vi "표지판 가공.vi"(1 "Paramaters":T4 {"Preprocessing Options"."Deviation Factor" min=0.0; "Preprocessing Options"."Threshold Limits"."Upper value" format="%.2f"; "Preprocessing Options"."Threshold Limits"."Lower value" format="%.2f"; "Preprocessing Options"."Threshold Range"."Upper value" format="%.2f"; "Preprocessing Options"."Threshold Range"."Lower value" format="%.2f"; "Preprocessing Options"."# of Erosions" min=0; "Preprocessing Options"."Method" items=["Manual Threshold"=-1, "-"=-2, "Auto Threshold: Clustering"=0, "Auto Threshold: Entropy"=1, "Auto Threshold: Metric"=2, "Auto Threshold: Moments"=3, "Auto Threshold: Inter-class Variance"=4, "--"=-3, "Local Threshold: Niblack"=5, "Local Threshold: BG Correction"=6]; "Preprocessing Options"."Looking for" items=["Bright Objects", "Dark Objects"]; "Nearest Neighbor Options"."Method" items=["Nearest Neighbor", "K Nearest Neighbor", "Minimum Mean Distance"]; "Nearest Neighbor Options"."Metric" items=["Maximum", "Sum", "Euclidean"]; "Nearest Neighbor Options"."k" min=3}, 2 "File Path":path=path "C:/Users/SeongHyeon/Desktop/[Github]_GPS Team/labview_program/작업중인 모든 Vi, dll파일 모음/전체프로그램/Sub Vi/Sensor/Vision Reference/곡선2.clf", 3 "Classifier Session (optional)":T2, 4 "Image 2":T1) -> (0 "주차냐":bool)   [LabVIEW 2016]
uses:
  <vilib>/vision/Classification.llb/IMAQ Classifier Nearest Neighbor options.ctl
  <vilib>/vision/Classification.llb/IMAQ Classifier Session.ctl
  <vilib>/vision/Image Controls.llb/IMAQ Image.ctl
  <vilib>/vision/NI_Vision_Development_Module.lvlib
panel:
  out "Identification Score":sgl
  out "Image":T1(plugin-control)
  in  "ROI Descriptor (Particle Classification 1)":T5={"Global Rectangle"=[693, 212, 1098, 745], "Contours"=[{"ID"=enum."External", "Type"=3, "Coordinates"=[693, 212, 1098, 745]}]} {"Contours"."Type" items=["No Selection", "Point", "Line", "Rectangle", "Oval", "Polygon", "Freehand Region", "Annulus", "Unused2", "Unused3", "Broken Line", "Freehand Line", "Rotated Rectangle"]}
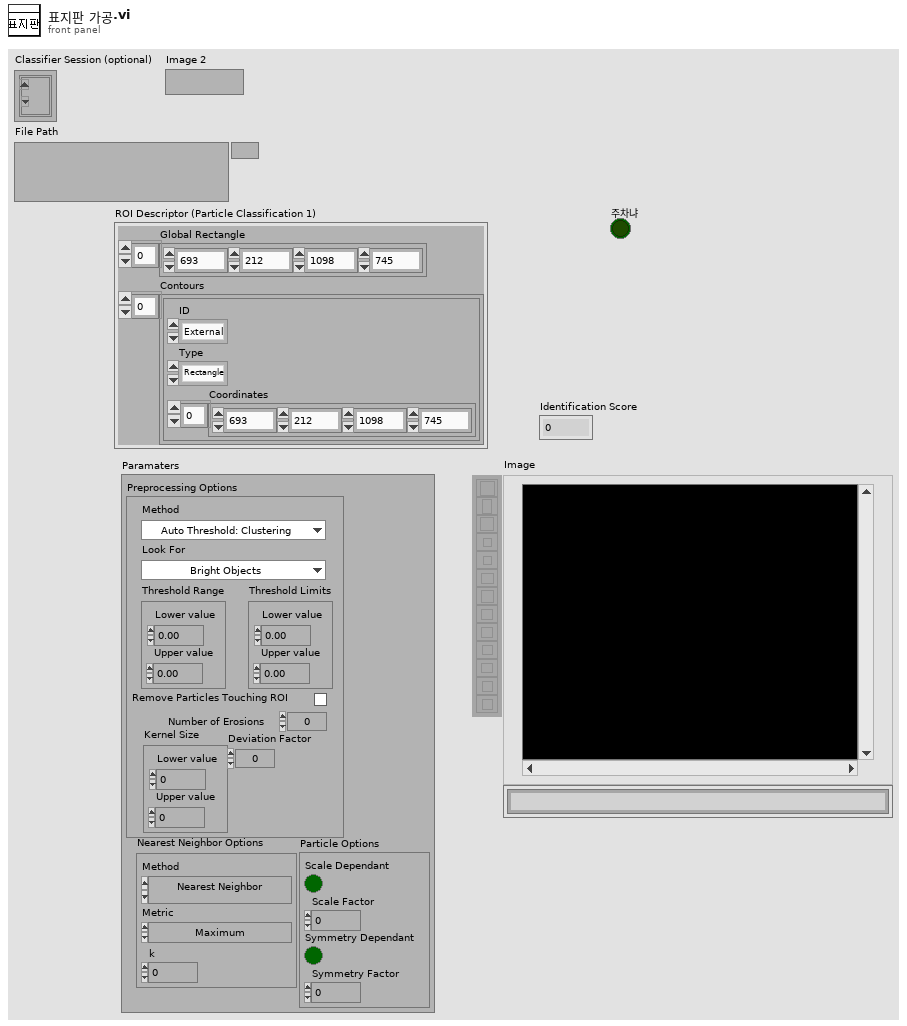
[diagram p1: front panel]
types:
  T1 = typedef "IMAQ Image.ctl" = refnum<image>
  T2 = typedef "IMAQ Classifier Session.ctl" = refnum<k1>
  T3 = typedef "IMAQ Classifier Nearest Neighbor options.ctl" = cluster{"Method":i32, "Metric":i32, "k":i32}
  T4 = cluster{"Preprocessing Options":cluster{"Method":i32, "Looking for":i32, "Threshold Range":cluster{"Lower value":sgl, "Upper value":sgl}, "Threshold Limits":cluster{"Lower value":sgl, "Upper value":sgl}, "Reject Border":bool, "# of Erosions":i32, "Kernel Size":cluster{"Lower value":i32, "Upper value":i32}, "Deviation Factor":dbl}, "Nearest Neighbor Options":T3, "Particle Options":cluster{"Scale Dependant":bool, "Scale Factor":sgl, "Symmetry Dependant":bool, "Symmetry Factor":sgl}}
  T5 = cluster{"Global Rectangle":i32[], "Contours":cluster{"ID":enum32{"External", "Internal"}, "Type":u32, "Coordinates":i32[]}[]}
  T6 = cluster{"Classification Score":sgl, "Identification Score":sgl}
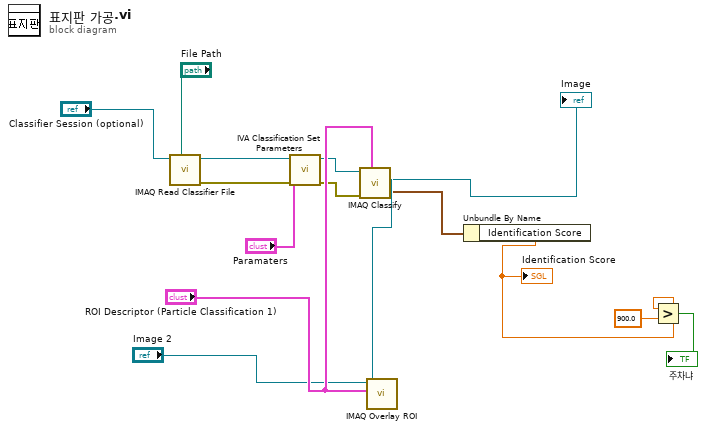
[diagram p0: block diagram]
diagram:
  n1 = call "IMAQ Read Classifier File"("File Path"="File Path", "Classifier Session (optional)"="Classifier Session (optional)") -> ("error out"=w11:errorcluster, "Classifier Session"=w12:T2)  [unwired: 5 in, 3 out]
  n2 = call <vilib>:"IVA Classification Set Parameters.vi"("error in"=w11, "Paramaters"="Paramaters", "Classifier Session In"=w12) -> ("error out"=w10:errorcluster, "Classifier Session Out"=w6:T2)  [unwired: 7 out]
  n3 = call "IMAQ Overlay ROI"("ROI Descriptor"="ROI Descriptor (Particle Classification 1)", "Image"="Image 2") -> ("Image Out"=w15:T1)  [unwired: 8 in, 1 out]
  n4 = call "IMAQ Classify"("ROI Descriptor"="ROI Descriptor (Particle Classification 1)", "error in (no error)"=w10, "Image"=w15, "Classifier Session"=w6) -> ("Image (dup)"=→"Image":T1, "Scores"=w13:T6)  [unwired: 2 in, 4 out]
  n5 = Unbundle By Name(w13) -> ("Identification Score"=w9:sgl)
  "Identification Score" <- w9
  n6 = Greater?(x=w9, y=sgl 900.0) -> (0:→"주차냐":bool)
